vi "List All Item Names.vi"(8 "error in (no error)":errorcluster, 11 "LookupTable Reference":refnum<data-value>) -> (0 "error out":errorcluster, 1 "None Found?":bool, 2 "All Items":string[](array[string]), 3 "LookupTable Reference Out":refnum<data-value>)   [LabVIEW 2019, in "LookupTable.lvlib" / "LookupTable.lvclass"]
uses:
  <vilib>/gpm_packages/@cs/lookup-table/Source/LookupTable/LookupTable.lvclass
  <vilib>/gpm_packages/@cs/lookup-table/Source/LookupTable/LookupTable.lvclass/LookupTable.ctl
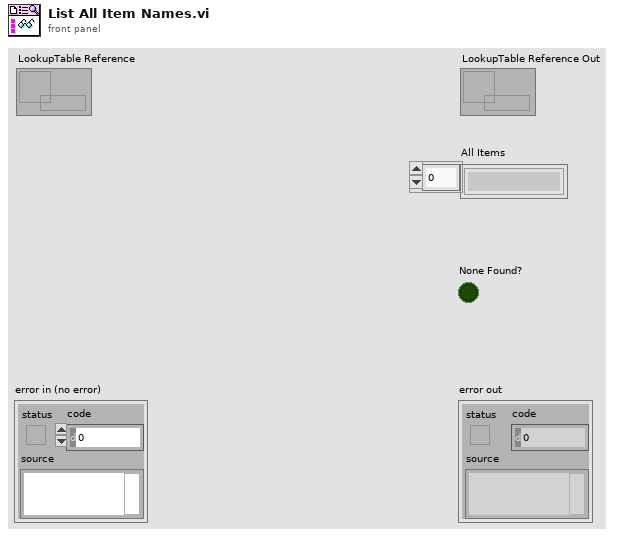
[diagram p1: front panel]
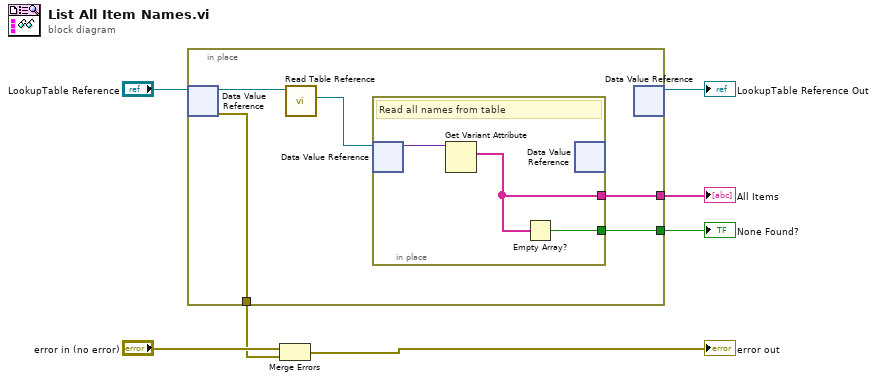
[diagram p0: block diagram]
diagram:
  n1 = in-place {
    in-place-border: [w12] -> w6
    in-place-border: [w11] -> w1
    in-place-border: [w10] -> w3
    n2 = in-place-dvr #1("LookupTable Reference") -> (w9:refnum<class "LookupTable.lvclass">, w10:errorcluster)
    n3 = call <vilib>:"Read Table Reference.vi"("LookupTable in"=w9) -> ("Table Reference"=w8:refnum<data-value>)  [unwired: 9 in, 1 out]
    n4 = in-place {
      in-place-border: [w14] -> w11
      in-place-border: [w15] -> w12
      # "Read all names from table"
      n5 = in-place-dvr #2(w8) -> (w13:variant)  [unwired: 1 out]
      n6 = Get Variant Attribute(Variant=w13) -> (names=w14:string[])  [unwired: 3 in, 3 out]
      n7 = Empty Array?(array=w14) -> (empty?=w15:bool)
      n8 = in-place-dvr #2() -> ()  [unwired: 1 in, 2 out]
    }
    n9 = in-place-dvr #1() -> (→"LookupTable Reference Out":refnum<data-value>)  [unwired: 1 in, 1 out]
  }
  "None Found?" <- w6
  "All Items" <- w1
  n10 = Merge Errors("error in (no error)", w3) -> (→"error out":errorcluster)
